vi "Write Channel Active.vi"(8 "error in":errorcluster, 10 "Channel Active":bool, 11 "Output Channels in":refnum<class "Output Channels.lvclass">) -> (0 "error out":errorcluster, 3 "Output Channels out":refnum<class "Output Channels.lvclass">)   [LabVIEW 2020, in "Plugin.lvlib" / "Output Channels.lvclass"]
doc: "Writes Channel Active."
uses:
  Output Channels.lvclass
  Output Channels.lvclass/Output Channels.ctl
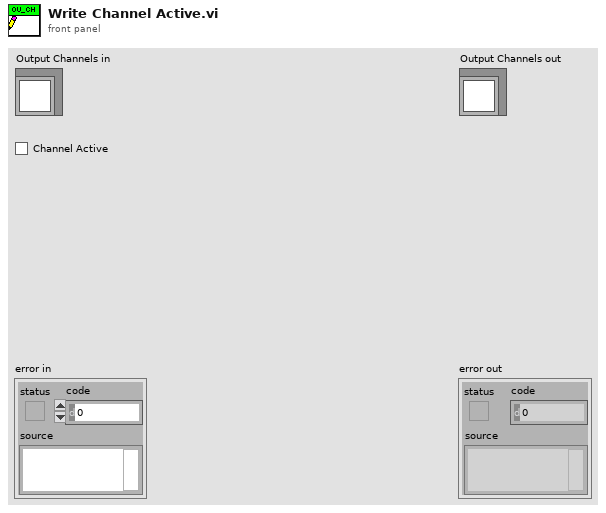
[diagram p1: front panel]
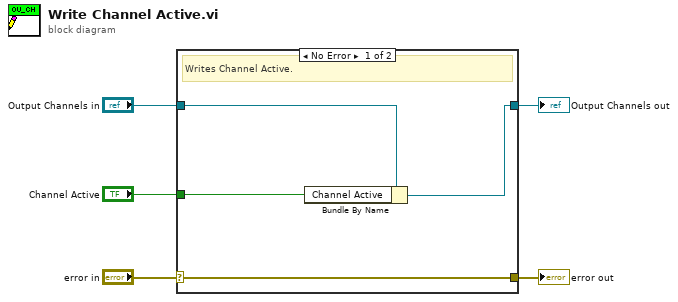
[diagram p0: block diagram]
diagram:
  n1 = case shown="No Error" "error in" {
    selector: "error in" -> [w9 w10]
    tunnel: [w9 w10] -> w4
    tunnel: [w7 w11] -> w2
    tunnel: "Output Channels in" -> [w8 w11]
    tunnel: "Channel Active" -> [w6 _]
    frame No Error {
      # "Writes Channel Active."
      n2 = Bundle By Name(cluster=w8, "Channel Active"=w6) -> (w7:refnum<class "Output Channels.lvclass">)
    }
    frame Error {
      # "Error"
    }
  }
  "error out" <- w4
  "Output Channels out" <- w2
